vi "Update.vi"(8 "error in":errorcluster, 11 "Cobra GUI in":refnum<class "Cobra GUI.lvclass">) -> (0 "error out":errorcluster, 3 "Cobra GUI out":refnum<class "Cobra GUI.lvclass">)   [LabVIEW 2019, in "Cobra GUI.lvlib" / "Cobra GUI.lvclass"]
uses:
  Cobra GUI.lvclass
  GUI 1.0/Controls/Module Graphs.ctl
  GUI 1.0/GUI.lvlib
  GUI 1.0/Controls/System Graphs.ctl
  GUI 1.0/Controls/Gauge Graphs/Current.ctl
  GUI 1.0/Controls/Gauge Graphs/Superheat.ctl
  GUI 1.0/Controls/Gauge Graphs/Subcooling.ctl
  GUI 1.0/Controls/Gauge Graphs/Compression Ratio.ctl
  GUI 1.0/Controls/Dial Gauges.ctl
  07690957-dc4f-472d-b35f-df7a883bd9a6.vi
  4b12478f-287d-4315-ba79-d40235526ef4.vi
  Private Controls/Module Command.ctl
  2d39f8a6-1858-4a68-ac92-16f5d1316896.vi
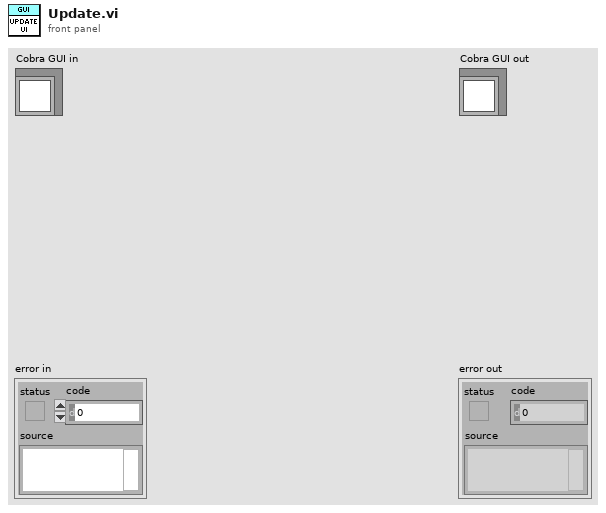
[diagram p1: front panel]
types:
  T1 = typedef "GUI.lvlib/System Graphs.ctl" = cluster{"Ambient Temp":dbl, "Suction Temp":dbl, "Condensor Temp":dbl, "Discharge Temp":dbl, "Bypass Steps":dbl}
  T2 = cluster{"M2 Thermal State":enum16{"Ramp Up", "Ramp Down", "Steady State", "Ebb and Flow", "Up", "Under Load", "Cryo Mode", "Shuttle Mode"}, "M1 Thermal State":enum16{"Ramp Up", "Ramp Down", "Steady State", "Ebb and Flow", "Up", "Under Load", "Cryo Mode"}, "High Side RPM":dbl, "Low Side RPM":dbl}
  T3 = typedef "GUI.lvlib/Dial Gauges.ctl" = cluster{"Condensing Pressure(psi)":dbl, "Compression Ratio":T4, "Subcool":T5, "Superheat":T6, "Current(A)":T7, "Suction Pressure(psi)":dbl}
  T4 = typedef "GUI.lvlib/Compression Ratio.ctl" = dbl
  T5 = typedef "GUI.lvlib/Subcooling.ctl" = dbl
  T6 = typedef "GUI.lvlib/Superheat.ctl" = dbl
  T7 = typedef "GUI.lvlib/Current.ctl" = dbl
  T8 = cluster{"Serial Number":string, "Compressor Hours":dbl, "SOM Storage(MB)":dbl, "Memory Available":dbl, "CPU Usage":dbl, "Software Version":string, "SD card free space":dbl, "Comp Temp":dbl, "Sleep Timer":dbl, "Sleep":bool, "Boot Up Time":timestamp}
  T9 = cluster{"M2 Heater %":dbl, "M2 Actuated":bool, "M2 Error":bool, "M2 Thermal Status":enum16{"Ramp Up", "Ramp Down", "Steady State", "Ebb and Flow", "Up", "Under Load", "Cryo Mode"}, "M2 Head State":enum16{"Disabled", "Run", "Error"}, "M2 Buffer":dbl, "M2 Valve Output":dbl}
  T10 = cluster{"M1 Heater %":dbl, "M1 Actuated":bool, "M1 Error":bool, "M1 Thermal Status":enum16{"Ramp Up", "Ramp Down", "Steady State", "Ebb and Flow", "Up", "Under Load", "Cryo Mode"}, "M1 Head State":enum16{"Disabled", "Run", "Error"}, "M1 Buffer":dbl, "M1 Valve Output":dbl}
  T11 = cluster{"Condensing Pressure":dbl, "Suction Pressure":dbl, "Bypass steps":u16, "Operating Time":dbl, "SubCooling":dbl, "Superheat":dbl, "M1 Superheat":dbl, "M2 Superheat":dbl, "Autotune output":dbl, "M1 Testing Elapsed Time":dbl, "M2 Testing Elapsed Time":dbl, "M1 Valve Control Mode":u8, "System Amps":dbl, "Compressor Run Time":dbl, "SD card free Space":dbl, "Free Memory":dbl, "M1 Pressure Feedback":dbl, "M2 Pressure Feedback":dbl, "Compression Ratio":dbl, "Serial Number":dbl, "M1 AC Load V":dbl, "M1 AC Load W":dbl, "M1 DC Load W":dbl, "M1 RH":dbl, "RH Threshold":dbl}
  T12 = cluster{"Name":string, "Time Stamp":timestamp, "Code":string, "Source":string, "Value":dbl, "Boolean":bool, "String":string, "Error":bool, "Warning":bool, " Fault":bool}[]
  T13 = cluster{"High Stage manual speed control":bool, "Manual High stage frequency":dbl, "Low Stage manual speed control":bool, "Manual Low Stage frequency":dbl}
  T14 = enum16{"Sleeping", "Warming up", "Ready", "Testing", "Restless", "Idle", "Sleeping Fault", "warning"}
  T15 = cluster{"port ":u16, "remote address":string, "Connection timeout ms":i32, "Waiting for connection":bool, "Waiting for Command":bool, "timeout ms":i32}[]
  T16 = typedef "LabGUI.lvlib/Module Command.ctl" = cluster{"Set Temp":dbl[unit], "Read Temp":dbl[unit], "Package":u16, "Bin String":string, "M1 Enable":bool, "TSD":bool}
  T17 = typedef "GUI.lvlib/System Status.ctl" = cluster{"Power On Off":bool, "Discharge Temp":dbl, "Liquid Temp":dbl, "Suction Temp":dbl, "Ambient Temp":dbl, "Sleep":bool, "System Status":u16, "M1 Actuated":bool, "M2 Actuated":bool, "Sleep Timer":dbl, "M1 Bin":cluster{"Bin String":string, "Bin Color":u16}, "M2 Bin":cluster{"Bin String":string, "Bin Color":u16}, "Discharge Pressure":dbl, "Suction Pressure":dbl, "Compression Ratio":dbl, "Compressor Amps":dbl, "Compressor Hours":dbl, "Bypass Steps":u16, "SubCooling":dbl, "SuperHeat":dbl, "Serial Number":string, "EMO detected":bool, "EMO Tripped":bool, "Thermal cutoff":bool, "Thermal cutoff 2":bool, "High Pressure switch":bool, "Running Time":timestamp, "SOM Status":cluster{"Boot Up Time":timestamp, "Software Version":string, "CPU Usage":dbl, "Memory Available":dbl, "SD card free space":dbl, "SOM Storage":dbl}, "Cascade Extra":cluster{"Discharge Temp High Side":dbl, "Suction Temp High Side":dbl, "Liquid Temp High side":dbl, "Discharge Pressure 2":dbl, "Suction Pressure 2":dbl, "Low Side RPM":dbl, "High Side RPM":dbl}}
  T18 = typedef "GUI.lvlib/Module Status.ctl" = cluster{"Case Temp":dbl, "Evap Temp":dbl, "Heater %":dbl, "EEV Steps":u32, "Set Temp":dbl, "Feedback":u8, "Power Drive":bool, "Piston Volts":dbl, "Safe Temp":bool, "Power":bool, "Thermal State":u16, "Error":bool, "In tollerance":bool, "Head State":u16, "Piston Force":dbl, "Package":string, "Dynamic SV":dbl, "PV":dbl, "TSD Temp":dbl, "DC Load Watts":dbl, "AC Load Watts":dbl, "Intec Feedback":dbl}
  T19 = typedef "GUI.lvlib/Config Data.ctl" = cluster{"Packages":cluster{"DUT Force lbf":cluster{" 0":u32, " 1":u32, " 2":u32, "3":u32, "4":u32, "5":u32, " 6":u32, "7":u32, "8":u32, "9":u32}, "DUT Names":cluster{"0":string, "1":string, "2":string, "3":string, "4":string, "5":string, "6":string, "7":string, "8":string, "9":string}}, "Heater PID":cluster{"P":dbl, "I":dbl, "D":dbl}, "Piston Settings":cluster{"Forces Slope":dbl, "Forces Intercept":dbl, "Transition Force":dbl, "Up Force":dbl, "Diameter (mm)":dbl, "Delay (ms)":dbl, "Pressure Ramp Delay (ms)":dbl}, "Safe Temps":cluster{"Minimum":i32, "Enabled":bool, "Maximum":i32}, "System Settings":cluster{"Number of Heads":i32, "60Hz Power":bool, "FTC200":bool, "AutoStartup":bool, "Purge":bool, "Sensors":bool, "HandClamp":bool, "ATE":bool, "Benchtop":bool, "Production":bool, "Refrigerant":u16, "Handler":bool, "Shuttle":bool, "220V":bool, "Cascade":bool, "Suction Sensor":u16, "Discharge Sensor":u16}, "Stepper Settings ":cluster{"Microstepping":u16, "Velocity":u8}, "Set Point Range":cluster{"Max":dbl, "Min":dbl}, "Pedestal Check DeltaT":dbl, "Ramp Delta T":dbl, "Ramp-SS Threshold":dbl, "SS Tolerance":dbl, "EEV PID":cluster{"Ramp Up Target":dbl, "Ramp Down Target":dbl, "Steady State Target":dbl, "Output":cluster{"Max":dbl, "Min":dbl}, "EBB and Flow Temp TH":dbl, "Cryomode EEV Max":dbl, "Valve minimum opening ":dbl, "Ramp Up EEV Steps":dbl, "Ramp Down EEV Steps":dbl, "SS EEV Steps Reset":dbl, "EBB and Flow Tol":dbl, "Gains":cluster{"P":dbl, "I":dbl, "D":dbl}, "Dissabled Target":dbl, "CryoMode Gains":cluster{"P":dbl, "I":dbl, "D":dbl}, "M1 SuperHeat Setpoint":dbl, "M2 Gains":cluster{"P":dbl, "I":dbl, "D":dbl}, "Flow Curve":u16}, "Sleep Timeout":dbl, "Bypass Values":cluster{"Bypass Valve":bool, "Flow Curve":u16, "Output":cluster{"Max":u32, "Min":u32}, "Feedback":u16, "Cyth Bypass":bool, "PID":cluster{"P":dbl, "I":dbl, "D":dbl}, "Pressure setpoint":i16, "Cryo Temp":i16, "Superheat Setpoint":i16, "Cryo Setpoint":i16}, "Default Temp":dbl, "InTEC":cluster{"Enabled":bool, "IP":string, "Port":u16}, "M1 TSD":cluster{"Gain":dbl, "Offset":dbl, "V Offset ":dbl}, "M2 TSD":cluster{"Gain":dbl, "Offset":dbl, "V Offset ":dbl}, "M1 T-Case Calibration":cluster{"Gain":dbl, "Offset":dbl}, "M2 T-Case Calibration":cluster{"Gain":dbl, "Offset":dbl}, "Heater PID TSD":cluster{"P":dbl, "I":dbl, "D":dbl}, "M2 Heater PID":cluster{"P":dbl, "I":dbl, "D":dbl}}
  T20 = cluster{"Compressor:":refnum<vi>, "NS Connection":refnum<vi>, "M1 Graphs":refnum<vi>, "M1 Main Waveform":refnum<vi>, "M2 Main Waveform":refnum<vi>, "M1 State":refnum<vi>, "M2 State":refnum<vi>, "M1 Commands":refnum<vi>, "M2 Commands":refnum<vi>, "M2 Graphs":refnum<vi>, "System Graphs":refnum<vi>, "M1 Cluster":refnum<vi>, "M2 Cluster":refnum<vi>, "TCP Connections":refnum<vi>, "M1 Humidity":refnum<vi>, "RT Status":refnum<vi>, "M1 Safe Temp and Head State":refnum<vi>, "M2 Safe Temp and Head State":refnum<vi>, "M1 Power Drive":refnum<vi>, "M2 Power Drive":refnum<vi>, "Gauges":refnum<vi>, "Cascade Compressor controls":refnum<vi>, "TCP commands":refnum<vi>, "Errors":refnum<vi>, "RT Events":refnum<vi>, "System Cluster":refnum<vi>, "Power On-Off":refnum<vi>, "Thermal Info":refnum<vi>, "Connected System":refnum<vi>}
  T21 = cluster{"Set Temp":dbl, "Read Temp":dbl, "Package":string, "Force":dbl, "Feedback":u8}
  T22 = cluster{"Set Temp":dbl[unit], "Read Temp":dbl[unit], "Package":u16, "Bin String":string, "M Enable":bool, "TSD":bool}
  T23 = cluster{"0":string, "1":string, "2":string, "3":string, "4":string, "5":string, "6":string, "7":string, "8":string, "9":string}
  T24 = typedef "GUI.lvlib/Module Graphs.ctl" = cluster{"Case Temp":dbl, "Evap Temp":dbl, "Heater Power (%)":dbl, "EEV Steps":dbl, "AC Load(W)":dbl}
  T25 = cluster{"Heater %":dbl, "Actuated":bool, "Error":bool, "Thermal Status":enum16{"Ramp Up", "Ramp Down", "Steady State", "Ebb and Flow", "Up", "Under Load", "Cryo Mode"}, "Head State":enum16{"Disabled", "Run", "Error"}, "Buffer":dbl, "Valve Output":dbl}
  T26 = cluster{"Boot Up Time":timestamp, "Software Version":string, "CPU Usage":dbl, "Memory Available":dbl, "SD card free space":dbl, "SOM Storage":dbl}
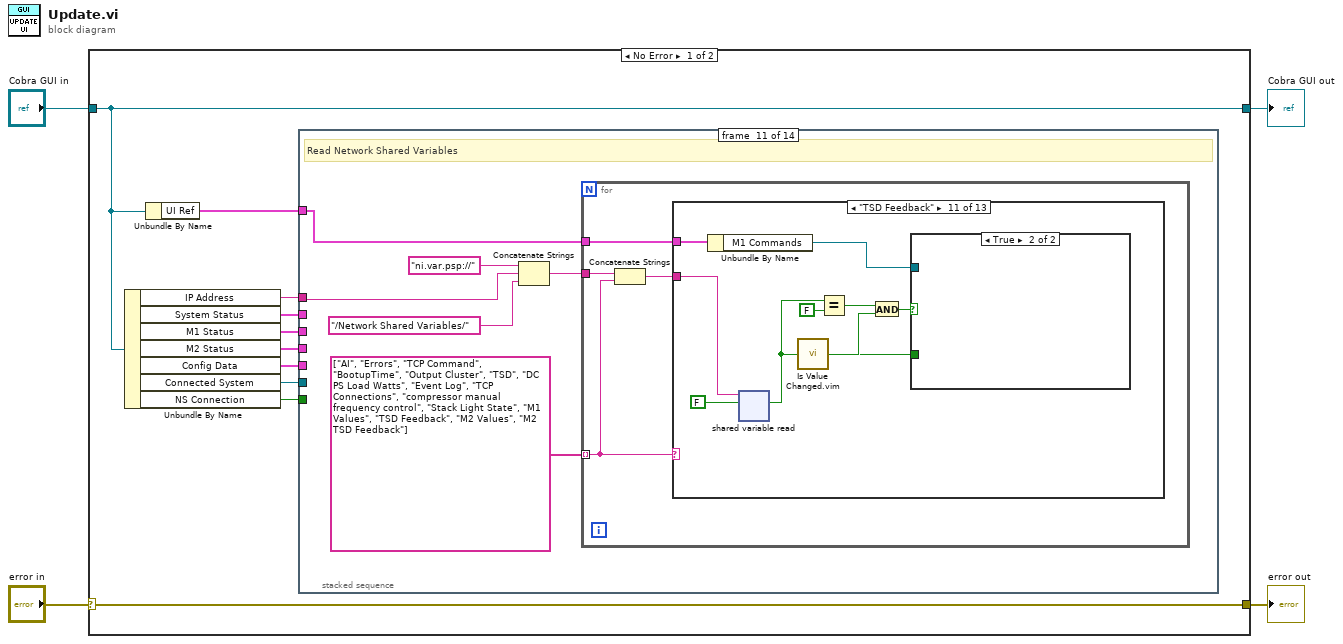
[diagram p0: block diagram]
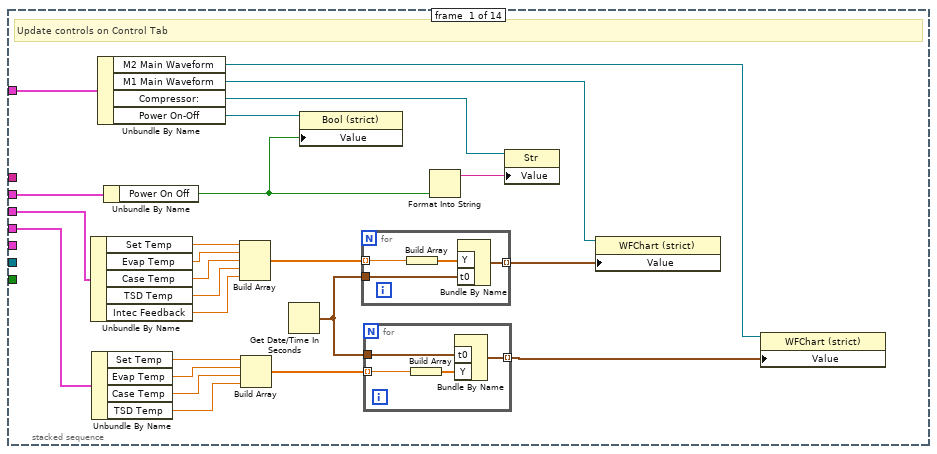
[diagram p2: hidden frame]
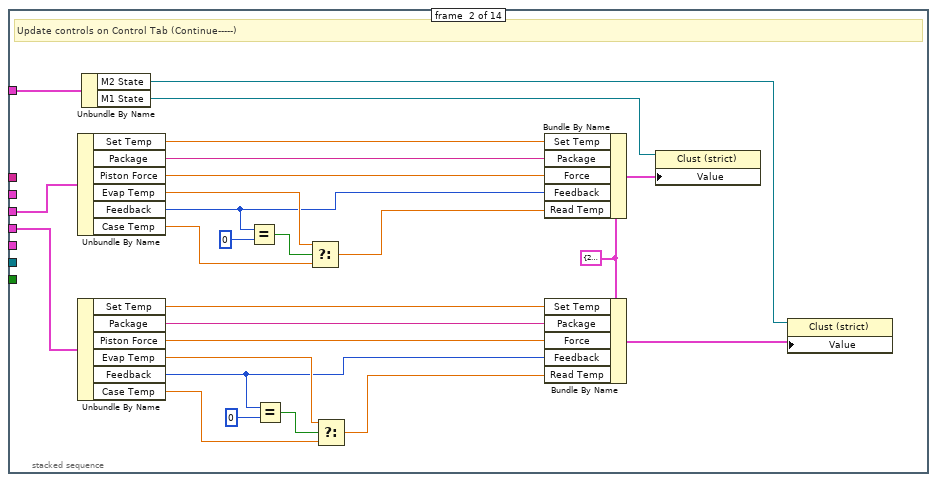
[diagram p3: hidden frame]
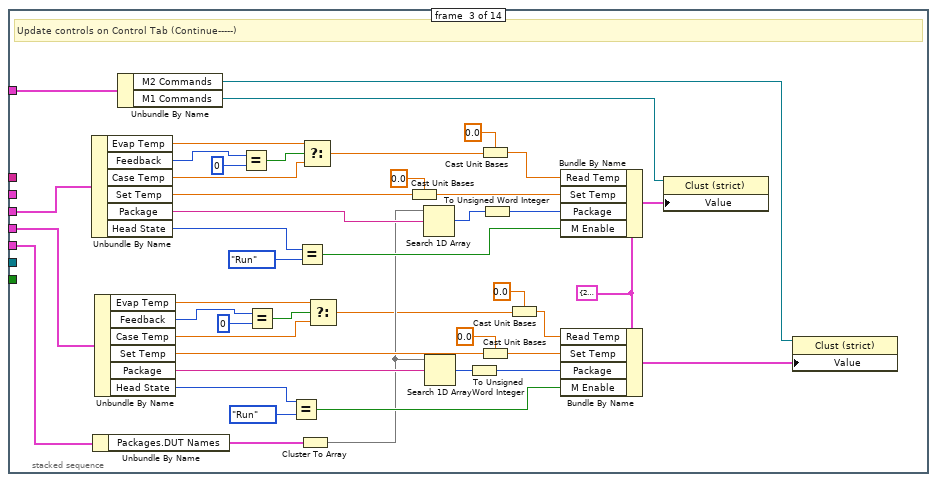
[diagram p4: hidden frame]
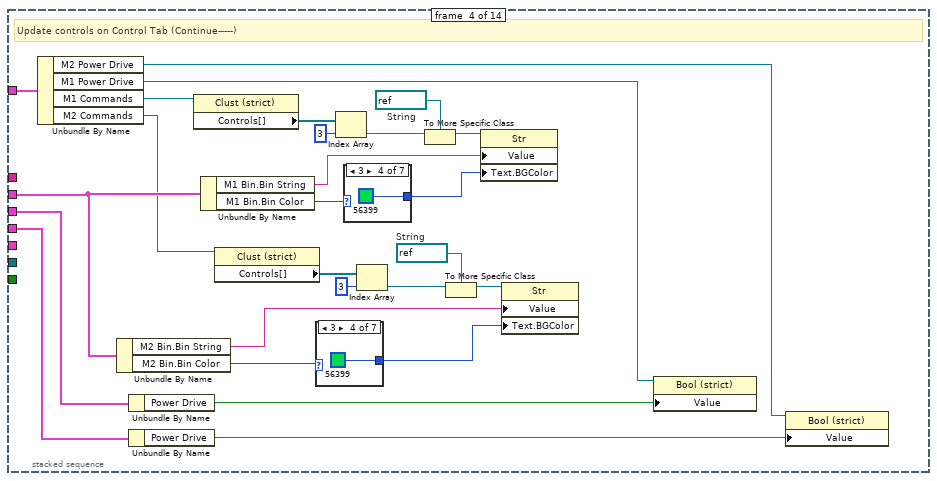
[diagram p5: hidden frame]
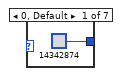
[diagram p6: hidden frame]
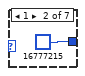
[diagram p7: hidden frame]
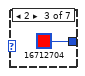
[diagram p8: hidden frame]
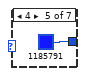
[diagram p9: hidden frame]
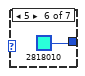
[diagram p10: hidden frame]
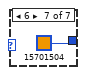
[diagram p11: hidden frame]
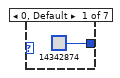
[diagram p12: hidden frame]
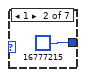
[diagram p13: hidden frame]
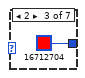
[diagram p14: hidden frame]
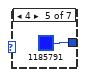
[diagram p15: hidden frame]
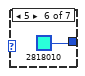
[diagram p16: hidden frame]
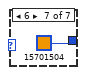
[diagram p17: hidden frame]
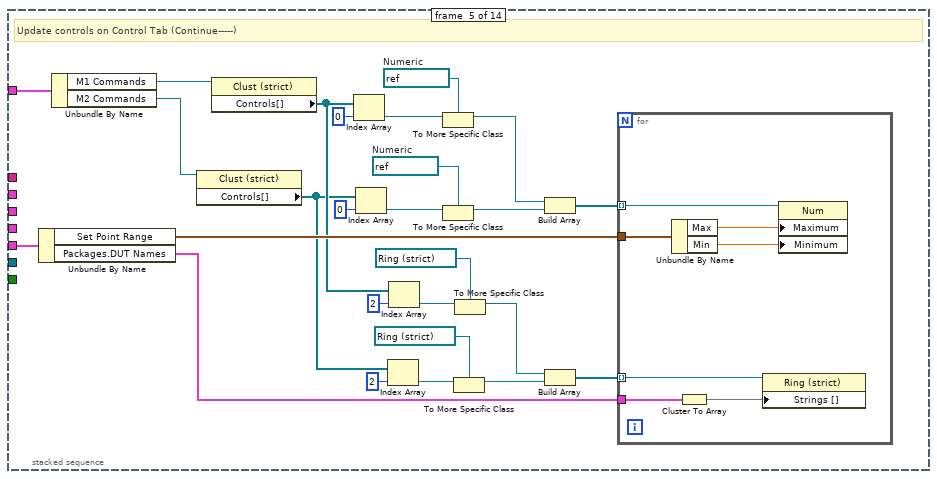
[diagram p18: hidden frame]
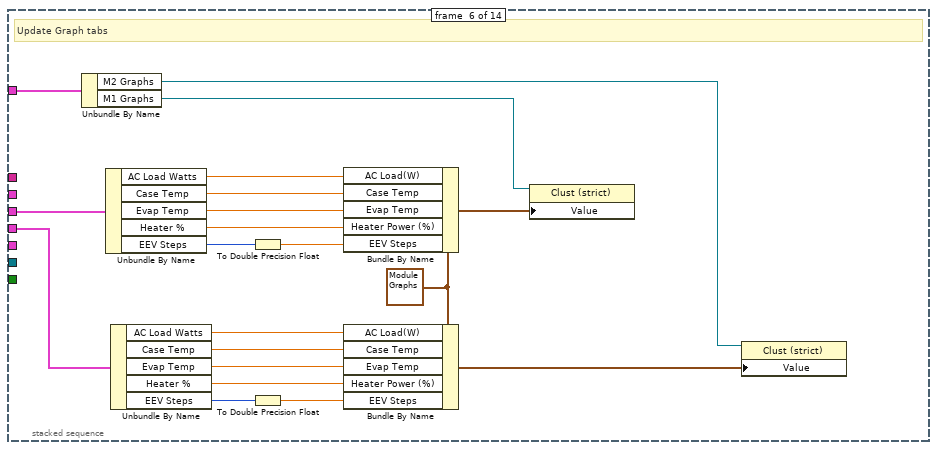
[diagram p19: hidden frame]
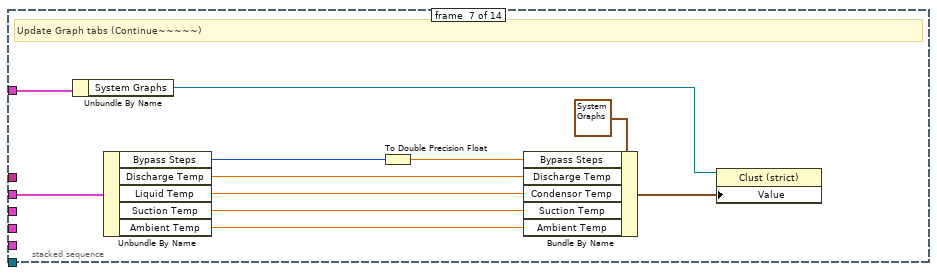
[diagram p20: hidden frame]
diagram:
  n1 = case shown="No Error" "error in" {
    selector: "error in" -> [w14 w440]
    tunnel: [w14 w440] -> w3
    tunnel: [w13 w439] -> w1
    tunnel: "Cobra GUI in" -> [w13 w439]
    frame No Error {
      n2 = Unbundle By Name(w13) -> ("IP Address"=w12:string, "System Status"=w11:T17, "M1 Status"=w10:T18, "M2 Status"=w9:T18, "Config Data"=w8:T19, "Connected System"=w7:refnum<vi>, "NS Connection"=w6:bool)
      n3 = Unbundle By Name(w13) -> ("UI Ref"=w5:T20)
      n4 = stacked-sequence {
        tunnel: w12 -> [_ _ _ _ _ _ _ _ _ _ w299 _ _ _]
        tunnel: w11 -> [w19 _ _ w143 _ _ w214 w229 w253 w292 _ _ _ w438]
        tunnel: w10 -> [w26 w57 w96 w142 _ w196 _ w228 w252 _ _ w411 _ _]
        tunnel: w9 -> [w25 w56 w95 w141 _ w195 _ w227 w251 _ _ _ w412 _]
        tunnel: w8 -> [_ _ w94 _ w183 _ _ _ _ _ _ w405 w419 w437]
        tunnel: w7 -> [_ _ _ _ _ _ _ _ _ _ _ _ _ _]
        tunnel: w6 -> [_ _ _ _ _ _ _ _ _ _ _ _ _ _]
        tunnel: w5 -> [w24 w55 w93 w140 w182 w197 w213 w226 w250 w279 w296 w410 w424 w431]
        frame #0 {
          # "Update controls on Control Tab"
          n5 = Unbundle By Name(w26) -> ("Set Temp"=w28:dbl, "Evap Temp"=w29:dbl, "Case Temp"=w30:dbl, "TSD Temp"=w31:dbl, "Intec Feedback"=w32:dbl)
          n6 = Unbundle By Name(w25) -> ("Set Temp"=w34:dbl, "Evap Temp"=w35:dbl, "Case Temp"=w36:dbl, "TSD Temp"=w37:dbl)
          n7 = Unbundle By Name(w24) -> ("M2 Main Waveform"=w20:refnum<vi>, "M1 Main Waveform"=w23:refnum<vi>, "Compressor:"=w18:refnum<vi>, "Power On-Off"=w16:refnum<vi>)
          n8 = Unbundle By Name(w19) -> ("Power On Off"=w15:bool)
          n9 = Build Array(w28, w29, w30, w31, w32) -> (w33:dbl[])
          n10 = Build Array(w34, w35, w36, w37) -> (w38:dbl[])
          n11 = Get Date/Time In Seconds() -> (seconds since 1Jan1904=w27:timestamp)
          n12 = property class="Bool (strict)"(reference=w16, "Value"=w15) -> ()  [unwired: 1 in, 2 out]
          n13 = for {
            tunnel: [w42] -> w22 mode=indexing
            tunnel: w27 -> [w41]
            tunnel: w33 -> [w39] mode=indexing
            n14 = Build Array(w39) -> (w40:dbl[])
            n15 = Bundle By Name("Y"=w40, "t0"=w41) -> (w42:waveform(dbl))  [unwired: 1 in]
          }
          n16 = for {
            tunnel: w27 -> [w45]
            tunnel: [w46] -> w21 mode=indexing
            tunnel: w38 -> [w43] mode=indexing
            n17 = Build Array(w43) -> (w44:dbl[])
            n18 = Bundle By Name("t0"=w45, "Y"=w44) -> (w46:waveform(dbl))  [unwired: 1 in]
          }
          n19 = Format Into String(w15) -> (resulting string=w17:string)  [unwired: 3 in, 1 out]
          n20 = property class="Str"(reference=w18, "Value"=w17) -> ()  [unwired: 1 in, 2 out]
          n21 = property class="WFChart (strict)"(reference=w23, "Value"=w22) -> ()  [unwired: 1 in, 2 out]
          n22 = property class="WFChart (strict)"(reference=w20, "Value"=w21) -> ()  [unwired: 1 in, 2 out]
        }
        frame #1 {
          w58 = T21 {"Set Temp"=20.0, "Read Temp"=0.0, "Package"="", "Force"=0.0, "Feedback"=1} ("M2 Data")
          # "Update controls on Control Tab (Continue-----)"
          n23 = Unbundle By Name(w57) -> ("Set Temp"=w59:dbl, "Package"=w60:string, "Piston Force"=w61:dbl, "Evap Temp"=w64:dbl, "Feedback"=w47:u8, "Case Temp"=w65:dbl)
          n24 = Unbundle By Name(w56) -> ("Set Temp"=w66:dbl, "Package"=w67:string, "Piston Force"=w68:dbl, "Evap Temp"=w72:dbl, "Feedback"=w49:u8, "Case Temp"=w71:dbl)
          n25 = Unbundle By Name(w55) -> ("M2 State"=w51:refnum<vi>, "M1 State"=w54:refnum<vi>)
          n26 = Equal?(x=w47, y=u8 0) -> (x = y?=w62:bool)
          n27 = Equal?(x=w49, y=u8 0) -> (x = y?=w70:bool)
          n28 = Select(t=w64, s=w62, f=w65) -> (s? t:f=w48:dbl)
          n29 = Select(t=w72, s=w70, f=w71) -> (s? t:f=w50:dbl)
          n30 = Bundle By Name(cluster=w58, "Set Temp"=w59, "Package"=w60, "Force"=w61, "Feedback"=w47, "Read Temp"=w48) -> (w53:T21)
          n31 = Bundle By Name(cluster=w58, "Set Temp"=w66, "Package"=w67, "Force"=w68, "Feedback"=w49, "Read Temp"=w50) -> (w52:T21)
          n32 = property on="Property Node" class="Clust (strict)"(reference=w54, "Value"=w53) -> ()  [unwired: 1 in, 2 out]
          n33 = property on="Property Node" class="Clust (strict)"(reference=w51, "Value"=w52) -> ()  [unwired: 1 in, 2 out]
        }
        frame #2 {
          w97 = T22 {"Set Temp"=273.15, "Read Temp"=273.15, "Package"=0, "Bin String"="", "M Enable"=TRUE, "TSD"=TRUE} ("M1 Commands")
          # "Update controls on Control Tab (Continue-----)"
          n34 = Unbundle By Name(w96) -> ("Evap Temp"=w82:dbl, "Feedback"=w83:u8, "Case Temp"=w84:dbl, "Set Temp"=w112:dbl, "Package"=w100:string, "Head State"=w103:u16)
          n35 = Unbundle By Name(w94) -> ("Packages.DUT Names"=w99:T23)
          n36 = Unbundle By Name(w95) -> ("Evap Temp"=w74:dbl, "Feedback"=w75:u8, "Case Temp"=w76:dbl, "Set Temp"=w115:dbl, "Package"=w101:string, "Head State"=w105:u16)
          n37 = Unbundle By Name(w93) -> ("M2 Commands"=w90:refnum<vi>, "M1 Commands"=w91:refnum<vi>)
          n38 = Equal?(x=w83, y=u8 0) -> (x = y?=w87:bool)
          n39 = Equal?(x=w75, y=u8 0) -> (x = y?=w78:bool)
          n40 = Equal?(x=w105, y=enum16{"Disabled", "Run", "Error"}."Run" ("Dataset.M1 Status.Head State")) -> (x = y?=w108:bool)
          n41 = Equal?(x=w103, y=enum16{"Disabled", "Run", "Error"}."Run" ("Dataset.M1 Status.Head State")) -> (x = y?=w111:bool)
          n42 = Cluster To Array(cluster=w99) -> (array=w98:string[])
          n43 = Select(t=w82, s=w87, f=w84) -> (s? t:f=w88:dbl)
          n44 = Select(t=w74, s=w78, f=w76) -> (s? t:f=w77:dbl)
          n45 = Cast Unit Bases(0:w112, 1:dbl[unit] 0.0 ("Set Temp")) -> (2:w113:dbl[unit])
          n46 = Search 1D Array(1D array=w98, element=w100) -> (index of element=w109:i32)  [unwired: 1 in]
          n47 = Search 1D Array(1D array=w98, element=w101) -> (index of element=w106:i32)  [unwired: 1 in]
          n48 = To Unsigned Word Integer(number=w106) -> (unsigned 16bit integer=w107:u16)
          n49 = Cast Unit Bases(0:w88, 1:dbl[unit] 0.0 ("Value")) -> (2:w81:dbl[unit])
          n50 = Cast Unit Bases(0:w115, 1:dbl[unit] 0.0 ("Set Temp")) -> (2:w117:dbl[unit])
          n51 = To Unsigned Word Integer(number=w109) -> (unsigned 16bit integer=w110:u16)
          n52 = Cast Unit Bases(0:w77, 1:dbl[unit] 0.0 ("Value")) -> (2:w73:dbl[unit])
          n53 = Bundle By Name(cluster=w97, "Read Temp"=w81, "Set Temp"=w113, "Package"=w110, "M Enable"=w111) -> (w92:T22)
          n54 = Bundle By Name(cluster=w97, "Read Temp"=w73, "Set Temp"=w117, "Package"=w107, "M Enable"=w108) -> (w89:T22)
          n55 = property on="Property Node" class="Clust (strict)"(reference=w91, "Value"=w92) -> ()  [unwired: 1 in, 2 out]
          n56 = property on="Property Node" class="Clust (strict)"(reference=w90, "Value"=w89) -> ()  [unwired: 1 in, 2 out]
        }
        frame #3 {
          w124 = refnum<vi> refnum  # String
          w130 = refnum<vi> refnum  # String
          # "Update controls on Control Tab (Continue-----)"
          n57 = Unbundle By Name(w140) -> ("M2 Power Drive"=w136:refnum<vi>, "M1 Power Drive"=w138:refnum<vi>, "M1 Commands"=w139:refnum<vi>, "M2 Commands"=w118:refnum<vi>)
          n58 = Unbundle By Name(w143) -> ("M2 Bin.Bin String"=w119:string, "M2 Bin.Bin Color"=w134:u16)
          n59 = Unbundle By Name(w142) -> ("Power Drive"=w137:bool)
          n60 = Unbundle By Name(w141) -> ("Power Drive"=w135:bool)
          n61 = property class="Clust (strict)"(reference=w139) -> ("Controls[]"=w133:refnum<vi>[])  [unwired: 1 in, 2 out]
          n62 = Unbundle By Name(w143) -> ("M1 Bin.Bin String"=w128:string, "M1 Bin.Bin Color"=w127:u16)
          n63 = property class="Clust (strict)"(reference=w118) -> ("Controls[]"=w121:refnum<vi>[])  [unwired: 1 in, 2 out]
          n64 = case shown="3" w134 {
            tunnel: [u32 14342874 u32 16777215 u32 16712704 u32 56399 u32 1185791 u32 2818010 u32 15701504] -> w120
            frame 0, Default {
            }
            frame 1 {
            }
            frame 2 {
            }
            frame 3 {
            }
            frame 4 {
            }
            frame 5 {
            }
            frame 6 {
            }
          }
          n65 = Index Array(array=w133, index=3) -> (element=w132:refnum<vi>)
          n66 = case shown="3" w127 {
            tunnel: [u32 14342874 u32 16777215 u32 16712704 u32 56399 u32 1185791 u32 2818010 u32 15701504] -> w126
            frame 0, Default {
            }
            frame 1 {
            }
            frame 2 {
            }
            frame 3 {
            }
            frame 4 {
            }
            frame 5 {
            }
            frame 6 {
            }
          }
          n67 = Index Array(array=w121, index=3) -> (element=w122:refnum<vi>)
          n68 = To More Specific Class(target class=w130, reference=w132) -> (specific class reference=w129:refnum<vi>)  [unwired: 1 in, 1 out]
          n69 = To More Specific Class(target class=w124, reference=w122) -> (specific class reference=w125:refnum<vi>)  [unwired: 1 in, 1 out]
          n70 = property class="Str"(reference=w129, "Value"=w128, "Text.BGColor"=w126) -> ()  [unwired: 1 in, 2 out]
          n71 = property class="Str"(reference=w125, "Value"=w119, "Text.BGColor"=w120) -> ()  [unwired: 1 in, 2 out]
          n72 = property class="Bool (strict)"(reference=w138, "Value"=w137) -> ()  [unwired: 1 in, 2 out]
          n73 = property class="Bool (strict)"(reference=w136, "Value"=w135) -> ()  [unwired: 1 in, 2 out]
        }
        frame #4 {
          w169 = refnum<vi> refnum  # Numeric
          w176 = refnum<vi> refnum  # Numeric
          # "Update controls on Control Tab (Continue-----)"
          n74 = Unbundle By Name(w183) -> ("Set Point Range"=w181:cluster{"Max":dbl, "Min":dbl}, "Packages.DUT Names"=w180:T23)
          n75 = Unbundle By Name(w182) -> ("M1 Commands"=w177:refnum<vi>, "M2 Commands"=w175:refnum<vi>)
          n76 = property class="Clust (strict)"(reference=w175) -> ("Controls[]"=w160:refnum<vi>[])  [unwired: 1 in, 2 out]
          n77 = property class="Clust (strict)"(reference=w177) -> ("Controls[]"=w166:refnum<vi>[])  [unwired: 1 in, 2 out]
          n78 = Index Array(array=w166, index=0) -> (element=w179:refnum<vi>)
          n79 = Index Array(array=w160, index=0) -> (element=w173:refnum<vi>)
          n80 = Index Array(array=w160, index=2) -> (element=w162:refnum<vi>)
          n81 = Index Array(array=w166, index=2) -> (element=w167:refnum<vi>)
          n82 = To More Specific Class(target class=w176, reference=w179) -> (specific class reference=w172:refnum<vi>)  [unwired: 1 in, 1 out]
          n83 = To More Specific Class(target class=w169, reference=w173) -> (specific class reference=w171:refnum<vi>)  [unwired: 1 in, 1 out]
          n84 = To More Specific Class(target class=refnum<vi> refnum ("Package"), reference=w162) -> (specific class reference=w159:refnum<vi>)  [unwired: 1 in, 1 out]
          n85 = To More Specific Class(target class=refnum<vi> refnum ("Package"), reference=w167) -> (specific class reference=w164:refnum<vi>)  [unwired: 1 in, 1 out]
          n86 = Build Array(w172, w171) -> (w170:refnum<vi>[])
          n87 = Build Array(w164, w159) -> (w158:refnum<vi>[])
          n88 = for {
            tunnel: w170 -> [w188] mode=indexing
            tunnel: w181 -> [w187]
            tunnel: w180 -> [w185]
            tunnel: w158 -> [w186] mode=indexing
            n89 = Unbundle By Name(w187) -> ("Max"=w189:dbl, "Min"=w190:dbl)
            n90 = Cluster To Array(cluster=w185) -> (array=w184:string[])
            n91 = property class="Ring (strict)"(reference=w186, "Strings []"=w184) -> ()  [unwired: 1 in, 2 out]
            n92 = property class="Num"(reference=w188, "Maximum"=w189, "Minimum"=w190) -> ()  [unwired: 1 in, 2 out]
          }
        }
        frame #5 {
          w210 = T24 {"Case Temp"=24.9375, "Evap Temp"=24.8046875, "Heater Power (%)"=0.0, "EEV Steps"=0.0, "AC Load(W)"=10.492394664499656} ("M1 Graphs")
          # "Update Graph tabs"
          n93 = Unbundle By Name(w197) -> ("M2 Graphs"=w192:refnum<vi>, "M1 Graphs"=w194:refnum<vi>)
          n94 = Unbundle By Name(w196) -> ("AC Load Watts"=w198:dbl, "Case Temp"=w199:dbl, "Evap Temp"=w200:dbl, "Heater %"=w201:dbl, "EEV Steps"=w202:u32)
          n95 = Unbundle By Name(w195) -> ("AC Load Watts"=w204:dbl, "Case Temp"=w205:dbl, "Evap Temp"=w206:dbl, "Heater %"=w207:dbl, "EEV Steps"=w208:u32)
          n96 = To Double Precision Float(number=w202) -> (double precision float=w203:dbl)
          n97 = To Double Precision Float(number=w208) -> (double precision float=w209:dbl)
          n98 = Bundle By Name(cluster=w210, "AC Load(W)"=w198, "Case Temp"=w199, "Evap Temp"=w200, "Heater Power (%)"=w201, "EEV Steps"=w203) -> (w193:T24)
          n99 = Bundle By Name(cluster=w210, "AC Load(W)"=w204, "Case Temp"=w205, "Evap Temp"=w206, "Heater Power (%)"=w207, "EEV Steps"=w209) -> (w191:T24)
          n100 = property class="Clust (strict)"(reference=w194, "Value"=w193) -> ()  [unwired: 1 in, 2 out]
          n101 = property class="Clust (strict)"(reference=w192, "Value"=w191) -> ()  [unwired: 1 in, 2 out]
        }
        frame #6 {
          # "Update Graph tabs (Continue~~~~~)"
          n102 = Unbundle By Name(w213) -> ("System Graphs"=w212:refnum<vi>)
          n103 = Unbundle By Name(w214) -> ("Bypass Steps"=w216:u16, "Discharge Temp"=w218:dbl, "Liquid Temp"=w219:dbl, "Suction Temp"=w220:dbl, "Ambient Temp"=w221:dbl)
          n104 = To Double Precision Float(number=w216) -> (double precision float=w217:dbl)
          n105 = Bundle By Name(cluster=T1 {"Ambient Temp"=77.534379824996, "Suction Temp"=77.78750485181808, "Condensor Temp"=77.29531729966402, "Discharge Temp"=78.09687988460064, "Bypass Steps"=72.0} ("System Graphs"), "Bypass Steps"=w217, "Discharge Temp"=w218, "Condensor Temp"=w219, "Suction Temp"=w220, "Ambient Temp"=w221) -> (w211:T1)
          n106 = property class="Clust (strict)"(reference=w212, "Value"=w211) -> ()  [unwired: 1 in, 2 out]
        }
        frame #7 {
          # "Update Graph tabs (Continue~~~~~)"
          n107 = Unbundle By Name(w226) -> ("Thermal Info"=w223:refnum<vi>, "Gauges"=w225:refnum<vi>)
          n108 = Unbundle By Name(w229) -> ("Compression Ratio"=w231:dbl, "Compressor Amps"=w232:dbl, "Discharge Pressure"=w233:dbl, "Suction Pressure"=w234:dbl, "SubCooling"=w235:dbl, "SuperHeat"=w236:dbl, "Cascade Extra.High Side RPM"=w240:dbl, "Cascade Extra.Low Side RPM"=w241:dbl)
          n109 = Unbundle By Name(w228) -> ("Thermal State"=w238:u16)
          n110 = Unbundle By Name(w227) -> ("Thermal State"=w239:u16)
          n111 = Round To Nearest(number=w240) -> (nearest integer value=w242:dbl)
          n112 = Round To Nearest(number=w241) -> (nearest integer value=w243:dbl)
          n113 = Bundle By Name(cluster=T3 {"Condensing Pressure(psi)"=165.57116807812622, "Compression Ratio"=1.0119646390563775, "Subcool"=-0.3368072880168427, "Superheat"=1.4200558413526494, "Current(A)"=0.2333286882987343, "Suction Pressure(psi)"=163.4397897916897} ("Gauges"), "Compression Ratio"=w231, "Current(A)"=w232, "Condensing Pressure(psi)"=w233, "Suction Pressure(psi)"=w234, "Subcool"=w235, "Superheat"=w236) -> (w224:T3)
          n114 = Bundle By Name(cluster=T2 {"M2 Thermal State"=enum."Ramp Up", "M1 Thermal State"=enum."Steady State", "High Side RPM"=0.0, "Low Side RPM"=0.0} ("Thermal Info"), "High Side RPM"=w242, "Low Side RPM"=w243, "M1 Thermal State"=w238, "M2 Thermal State"=w239) -> (w222:T2)
          n115 = property class="Clust (strict)"(reference=w225, "Value"=w224) -> ()  [unwired: 1 in, 2 out]
          n116 = property class="Clust (strict)"(reference=w223, "Value"=w222) -> ()  [unwired: 1 in, 2 out]
        }
        frame #8 {
          w268 = T25 {"Heater %"=0.0, "Actuated"=FALSE, "Error"=FALSE, "Thermal Status"=enum."Steady State", "Head State"=enum."Disabled", "Buffer"=0.9999999999999998, "Valve Output"=0.0} ("M1 Cluster")
          # "Update Debug tab"
          n117 = Unbundle By Name(w250) -> ("M2 Cluster"=w245:refnum<vi>, "M1 Cluster"=w247:refnum<vi>, "System Cluster"=w249:refnum<vi>)
          n118 = Unbundle By Name(w253) -> ("Sleep"=w255:bool, "Sleep Timer"=w256:dbl, "Discharge Temp"=w257:dbl, "Compressor Hours"=w258:dbl, "Serial Number"=w259:string)
          n119 = Unbundle By Name(w252) -> ("Head State"=w260:u16, "Thermal State"=w261:u16, "Error"=w262:bool, "Heater %"=w263:dbl)
          n120 = Unbundle By Name(w251) -> ("Head State"=w264:u16, "Thermal State"=w265:u16, "Error"=w266:bool, "Heater %"=w267:dbl)
          n121 = Bundle By Name(cluster=T8 {"Serial Number"="204300076", "Compressor Hours"=59.65, "SOM Storage(MB)"=243.036, "Memory Available"=353.72, "CPU Usage"=40.953570959266244, "Software Version"="SW Version:CC 21.4.8.1", "SD card free space"=31.886, "Comp Temp"=78.09687988460064, "Sleep Timer"=-1.0, "Sleep"=TRUE, "Boot Up Time"=timestamp(3700144843.654765 s since 1904-01-01)} ("System Cluster"), "Sleep"=w255, "Sleep Timer"=w256, "Comp Temp"=w257, "Compressor Hours"=w258, "Serial Number"=w259) -> (w248:T8)
          n122 = Bundle By Name(cluster=w268, "Head State"=w260, "Thermal Status"=w261, "Error"=w262, "Heater %"=w263) -> (w246:T25)
          n123 = Bundle By Name(cluster=w268, "Head State"=w264, "Thermal Status"=w265, "Error"=w266, "Heater %"=w267) -> (w244:T25)
          n124 = property class="Clust (strict)"(reference=w249, "Value"=w248) -> ()  [unwired: 1 in, 2 out]
          n125 = property class="Clust (strict)"(reference=w247, "Value"=w246) -> ()  [unwired: 1 in, 2 out]
          n126 = property class="Clust (strict)"(reference=w245, "Value"=w244) -> ()  [unwired: 1 in, 2 out]
        }
        frame #9 {
          # "Update Debug tab (Continue~~~~)"
          n127 = Unbundle By Name(w279) -> ("System Cluster"=w278:refnum<vi>, "M2 Cluster"=w274:refnum<vi>, "M2 Cluster"=w272:refnum<vi>)
          n128 = Unbundle By Name(w292) -> ("M2 Actuated"=w269:bool, "M1 Actuated"=w273:bool, "SOM Status"=w280:T26)
          n129 = Unbundle By Name(w280) -> ("Memory Available"=w283:dbl, "SOM Storage"=w284:dbl, "SD card free space"=w285:dbl, "CPU Usage"=w290:dbl, "Software Version"=w291:string)
          n130 = Bundle By Name(cluster=T9 {"M2 Heater %"=0.0, "M2 Actuated"=FALSE, "M2 Error"=FALSE, "M2 Thermal Status"=enum."Steady State", "M2 Head State"=enum."Disabled", "M2 Buffer"=0.9999999999999998, "M2 Valve Output"=0.0} ("M2 Cluster"), "M2 Actuated"=w269) -> (w271:T9)
          n131 = property class="Clust (strict)"(reference=w272, "Value"=w271) -> ()  [unwired: 1 in, 2 out]
          n132 = Build Array(w283, w284, w285) -> (w282:dbl[])
          n133 = for {
            tunnel: w282 -> [w294] mode=indexing
            tunnel: [w293] -> w281 mode=indexing
            n134 = Divide(x=w294, y=1000.0) -> (x/y=w293:dbl)
          }
          n135 = Bundle By Name(cluster=T10 {"M1 Heater %"=0.0, "M1 Actuated"=FALSE, "M1 Error"=FALSE, "M1 Thermal Status"=enum."Ramp Up", "M1 Head State"=enum."Disabled", "M1 Buffer"=0.0, "M1 Valve Output"=0.0} ("Value"), "M1 Actuated"=w273) -> (w275:T10)
          n136 = Index Array(array=w281) -> (element #1=w287:dbl, element #2=w288:dbl, element #3=w289:dbl)  [unwired: 3 in]
          n137 = property class="Clust (strict)"(reference=w274, "Value"=w275) -> ()  [unwired: 1 in, 2 out]
          n138 = Bundle By Name(cluster=T8 {"Serial Number"="204300076", "Compressor Hours"=59.65, "SOM Storage(MB)"=243.036, "Memory Available"=353.72, "CPU Usage"=40.953570959266244, "Software Version"="SW Version:CC 21.4.8.1", "SD card free space"=31.886, "Comp Temp"=78.09687988460064, "Sleep Timer"=-1.0, "Sleep"=TRUE, "Boot Up Time"=timestamp(3700144843.654765 s since 1904-01-01)} ("System Cluster"), "Memory Available"=w287, "SOM Storage(MB)"=w288, "SD card free space"=w289, "CPU Usage"=w290, "Software Version"=w291) -> (w277:T8)
          n139 = property class="Clust (strict)"(reference=w278, "Value"=w277) -> ()  [unwired: 1 in, 2 out]
        }
        frame #10 {
          # "Read Network Shared Variables"
          n140 = Concatenate Strings("ni.var.psp://", w299, "/Network Shared Variables/") -> (w297:string)
          n141 = for {
            tunnel: string[] ["AI", "Errors", "TCP Command", "BootupTime", "Output Cluster", "TSD", "DC PS Load Watts", "Event Log", "TCP Connections", "compressor manual frequency control", "Stack Light State", "M1 Values", "TSD Feedback", "M2 Values", "M2 TSD Feedback"] -> [w304] mode=indexing
            tunnel: w297 -> [w305]
            tunnel: w296 -> [w302]
            n142 = Concatenate Strings(w305, w304) -> (w303:string)
            n143 = case shown="\"TSD Feedback\"" w304 {
              tunnel: w303 -> [w309 _ w318 w325 w330 w335 w340 w346 w356 w364 w373 w386 w395]
              tunnel: w302 -> [w308 _ w317 w324 w329 w334 w338 w344 w354 w363 w367 w380 w393]
              frame "Output Cluster" {
                n144 = Unbundle By Name(w308) -> ("M1 Humidity"=w307:refnum<vi>)
                n145 = shared-variable-read(w309, T11 {"Condensing Pressure"=0.0, "Suction Pressure"=0.0, "Bypass steps"=0, "Operating Time"=0.0, "SubCooling"=0.0, "Superheat"=0.0, "M1 Superheat"=0.0, "M2 Superheat"=0.0, "Autotune output"=0.0, "M1 Testing Elapsed Time"=0.0, "M2 Testing Elapsed Time"=0.0, "M1 Valve Control Mode"=0, "System Amps"=0.0, "Compressor Run Time"=0.0, "SD card free Space"=0.0, "Free Memory"=0.0, "M1 Pressure Feedback"=0.0, "M2 Pressure Feedback"=0.0, "Compression Ratio"=0.0, "Serial Number"=0.0, "M1 AC Load V"=0.0, "M1 AC Load W"=0.0, "M1 DC Load W"=0.0, "M1 RH"=0.0, "RH Threshold"=0.0} ("output cluster")) -> (w311:T11)  [unwired: 1 in, 3 out]
                n146 = Unbundle By Name(w311) -> ("RH Threshold"=w313:dbl, "M1 RH"=w312:dbl)
                n147 = Bundle("RH Threshold"=w313, "M1 RH"=w312) -> (w306:cluster{"RH Threshold":dbl, "M1 RH":dbl})  [unwired: 1 in]
                n148 = property class="WFChart (strict)"(reference=w307, "Value"=w306) -> ()  [unwired: 1 in, 2 out]
              }
              frame "TSD" {
              }
              frame "Event Log" {
                n149 = Unbundle By Name(w317) -> ("RT Events"=w314:refnum<vi>)
                n150 = shared-variable-read(w318, T12 [] ("Event Log")) -> (w315:T12)  [unwired: 1 in, 3 out]
                n151 = call "Is Value Changed.vim"("value"=w315) -> ("changed or first call?"=w316:bool)
                n152 = case shown="True" w316 {
                  tunnel: w315 -> [_ w321]
                  tunnel: w314 -> [_ w320]
                  frame False {
                  }
                  frame True {
                    n153 = property class="Arr (strict)"(reference=w320, "Value"=w321) -> ()  [unwired: 1 in, 2 out]
                  }
                }
              }
              frame "Errors" {
                n154 = Unbundle By Name(w324) -> ("Errors"=w323:refnum<vi>)
                n155 = shared-variable-read(w325, string[] [] ("Errors 2")) -> (w322:string[])  [unwired: 1 in, 3 out]
                n156 = property class="Arr (strict)"(reference=w323, "Value"=w322) -> ()  [unwired: 1 in, 2 out]
              }
              frame "TCP Command" {
                n157 = Unbundle By Name(w329) -> ("TCP commands"=w328:refnum<vi>)
                n158 = shared-variable-read(w330, string[] [] ("Errors 2")) -> (w327:string[])  [unwired: 1 in, 3 out]
                n159 = property class="Arr (strict)"(reference=w328, "Value"=w327) -> ()  [unwired: 1 in, 2 out]
              }
              frame "compressor manual frequency control" {
                n160 = Unbundle By Name(w334) -> ("Cascade Compressor controls"=w333:refnum<vi>)
                n161 = shared-variable-read(w335, T13 {"High Stage manual speed control"=FALSE, "Manual High stage frequency"=0.0, "Low Stage manual speed control"=FALSE, "Manual Low Stage frequency"=0.0} ("Cascade Compressor controls")) -> (w332:T13)  [unwired: 1 in, 3 out]
                n162 = property class="Clust (strict)"(reference=w333, "Value"=w332) -> ()  [unwired: 1 in, 2 out]
              }
              frame "Stack Light State" {
                n163 = Unbundle By Name(w338) -> ("RT Status"=w337:refnum<vi>)
                n164 = shared-variable-read(w340, T14."Sleeping Fault" ("Stack light states")) -> (w342:T14)  [unwired: 1 in, 3 out]
                n165 = Format Into String(w342) -> (resulting string=w339:string)  [unwired: 3 in, 1 out]
                n166 = property class="Str"(reference=w337, "Value"=w339) -> ()  [unwired: 1 in, 2 out]
              }
              frame "M1 Values" {
                n167 = Unbundle By Name(w344) -> ("M1 Cluster"=w343:refnum<vi>)
                n168 = shared-variable-read(w346, dbl[] [0.0, 0.0]) -> (w348:dbl[])  [unwired: 1 in, 3 out]
                n169 = Index Array(array=w348) -> (element #1=w350:dbl, element #2=w351:dbl)  [unwired: 2 in]
                n170 = Bundle By Name(cluster=T10 {"M1 Heater %"=0.0, "M1 Actuated"=FALSE, "M1 Error"=FALSE, "M1 Thermal Status"=enum."Steady State", "M1 Head State"=enum."Disabled", "M1 Buffer"=0.9999999999999998, "M1 Valve Output"=0.0} ("M1 Cluster"), "M1 Buffer"=w350, "M1 Valve Output"=w351) -> (w345:T10)
                n171 = property class="Clust (strict)"(reference=w343, "Value"=w345) -> ()  [unwired: 1 in, 2 out]
              }
              frame "M2 Values" {
                n172 = Unbundle By Name(w354) -> ("M2 Cluster"=w353:refnum<vi>)
                n173 = shared-variable-read(w356, dbl[] [0.0, 0.0]) -> (w358:dbl[])  [unwired: 1 in, 3 out]
                n174 = Index Array(array=w358) -> (element #1=w359:dbl, element #2=w360:dbl)  [unwired: 2 in]
                n175 = Bundle By Name(cluster=T9 {"M2 Heater %"=0.0, "M2 Actuated"=FALSE, "M2 Error"=FALSE, "M2 Thermal Status"=enum."Steady State", "M2 Head State"=enum."Disabled", "M2 Buffer"=0.9999999999999998, "M2 Valve Output"=0.0} ("M2 Cluster"), "M2 Buffer"=w359, "M2 Valve Output"=w360) -> (w355:T9)
                n176 = property class="Clust (strict)"(reference=w353, "Value"=w355) -> ()  [unwired: 1 in, 2 out]
              }
              frame "TCP Connections" {
                n177 = Unbundle By Name(w363) -> ("TCP Connections"=w361:refnum<vi>)
                n178 = shared-variable-read(w364, T15 [{"port "=1300, "remote address"="", "Connection timeout ms"=100, "Waiting for connection"=TRUE, "Waiting for Command"=TRUE, "timeout ms"=5000}] ("TCP Connections")) -> (w362:T15)  [unwired: 1 in, 3 out]
                n179 = property class="Arr (strict)"(reference=w361, "Value"=w362) -> ()  [unwired: 1 in, 2 out]
              }
              frame "TSD Feedback" {
                n180 = Unbundle By Name(w367) -> ("M1 Commands"=w366:refnum<vi>)
                n181 = shared-variable-read(w373, FALSE ("data type")) -> (w368:bool)  [unwired: 1 in, 3 out]
                n182 = call "Is Value Changed.vim"("value"=w368) -> ("changed or first call?"=w370:bool)
                n183 = Equal?(x=w368, y=FALSE) -> (x = y?=w369:bool)
                n184 = And(x=w369, y=w370) -> (x .and. y?=w372:bool)
                n185 = case shown="True" w372 {
                  tunnel: w368 -> [w376 _]
                  tunnel: w366 -> [w378 _]
                  frame False {
                    n186 = Bundle By Name(cluster=T16 {"Set Temp"=273.15, "Read Temp"=273.15, "Package"=0, "Bin String"="", "M1 Enable"=TRUE, "TSD"=TRUE} ("Value"), "TSD"=w376) -> (w375:T16)
                    n187 = property on="Property Node" class="Clust (strict)"(reference=w378, "Value"=w375) -> ()  [unwired: 1 in, 2 out]
                  }
                  frame True {
                  }
                }
              }
              frame "M2 TSD Feedback" {
                n188 = Unbundle By Name(w380) -> ("M2 Commands"=w379:refnum<vi>)
                n189 = shared-variable-read(w386, FALSE ("data type")) -> (w381:bool)  [unwired: 1 in, 3 out]
                n190 = call "Is Value Changed.vim"("value"=w381) -> ("changed or first call?"=w383:bool)
                n191 = Equal?(x=w381, y=FALSE) -> (x = y?=w382:bool)
                n192 = And(x=w382, y=w383) -> (x .and. y?=w385:bool)
                n193 = case shown="False" w385 {
                  tunnel: w381 -> [w389 _]
                  tunnel: w379 -> [w391 _]
                  frame False {
                    n194 = Bundle By Name(cluster=T16 {"Set Temp"=273.15, "Read Temp"=273.15, "Package"=0, "Bin String"="", "M1 Enable"=TRUE, "TSD"=TRUE} ("Value"), "TSD"=w389) -> (w388:T16)
                    n195 = property on="Property Node" class="Clust (strict)"(reference=w391, "Value"=w388) -> ()  [unwired: 1 in, 2 out]
                  }
                  frame True {
                  }
                }
              }
              frame "BootupTime", Default {
                n196 = Unbundle By Name(w393) -> ("System Cluster"=w392:refnum<vi>)
                n197 = shared-variable-read(w395, timestamp(0 s since 1904-01-01)) -> (w398:timestamp)  [unwired: 1 in, 3 out]
                n198 = Bundle By Name(cluster=T8 {"Serial Number"="204300076", "Compressor Hours"=59.65, "SOM Storage(MB)"=243.036, "Memory Available"=353.72, "CPU Usage"=40.953570959266244, "Software Version"="SW Version:CC 21.4.8.1", "SD card free space"=31.886, "Comp Temp"=78.09687988460064, "Sleep Timer"=-1.0, "Sleep"=TRUE, "Boot Up Time"=timestamp(3700144843.654765 s since 1904-01-01)} ("System Cluster"), "Boot Up Time"=w398) -> (w394:T8)
                n199 = property class="Clust (strict)"(reference=w392, "Value"=w394) -> ()  [unwired: 1 in, 2 out]
              }
            }
          }
        }
        frame #11 {
          # "Visibility of Controls (Continue~~~~~)"
          n200 = Unbundle By Name(w410) -> ("M1 Safe Temp and Head State"=w408:refnum<vi>, "M1 Power Drive"=w407:refnum<vi>)
          n201 = Unbundle By Name(w405) -> ("Piston Settings.Diameter (mm)"=w406:dbl, "Safe Temps.Enabled"=w402:bool)
          n202 = Unbundle By Name(w411) -> ("Safe Temp"=w401:bool, "Head State"=w409:u16)
          n203 = And(x=w402, y=w401) -> (x .and. y?=w399:bool)
          n204 = Equal To 0?(x=w409) -> (x = 0?=w404:bool)
          n205 = Greater Than 0?(x=w406) -> (x > 0?=w403:bool)
          n206 = And(x=w403, y=w399) -> (x .and. y?=w400:bool)
          n207 = property class="Bool (strict)"(reference=w407, "Visible"=w400) -> ()  [unwired: 1 in, 2 out]
          n208 = property class="Bool (strict)"(reference=w408, "Visible"=w399, "Value"=w404) -> ()  [unwired: 1 in, 2 out]
        }
        frame #12 {
          # "Visibility of Controls (Continue~~~~~)"
          n209 = Unbundle By Name(w424) -> ("M2 Safe Temp and Head State"=w422:refnum<vi>, "M2 Power Drive"=w421:refnum<vi>)
          n210 = Unbundle By Name(w419) -> ("Piston Settings.Diameter (mm)"=w420:dbl, "Safe Temps.Enabled"=w416:bool)
          n211 = Unbundle By Name(w412) -> ("Safe Temp"=w415:bool, "Head State"=w423:u16)
          n212 = And(x=w416, y=w415) -> (x .and. y?=w413:bool)
          n213 = Equal To 0?(x=w423) -> (x = 0?=w418:bool)
          n214 = Greater Than 0?(x=w420) -> (x > 0?=w417:bool)
          n215 = And(x=w417, y=w413) -> (x .and. y?=w414:bool)
          n216 = property class="Bool (strict)"(reference=w421, "Visible"=w414) -> ()  [unwired: 1 in, 2 out]
          n217 = property class="Bool (strict)"(reference=w422, "Visible"=w413, "Value"=w418) -> ()  [unwired: 1 in, 2 out]
        }
        frame #13 {
          w428 = refnum<vi> refnum  # Numeric
          n218 = Unbundle By Name(w431) -> ("Thermal Info"=w430:refnum<vi>)  [unwired: 1 out]
          n219 = Unbundle By Name(w437) -> ("System Settings.Cascade"=w435:bool)
          n220 = Unbundle By Name(w438) -> ("Compressor Amps"=w433:dbl, "Power On Off"=w434:bool)
          n221 = Round To Nearest(number=w433) -> (nearest integer value=w436:dbl)
          n222 = Not Equal To 0?(x=w436) -> (x != 0?=w432:bool)
          n223 = And(x=w432, y=w434) -> (x .and. y?=w425:bool)
          n224 = property class="Clust (strict)"(reference=w430) -> ("Controls[]"=w427:refnum<vi>[])  [unwired: 1 in, 2 out]
          n225 = And(x=w434, y=w435) -> ()  [unwired: 1 out]
          n226 = Index Array(array=w427) -> (element #1=w429:refnum<vi>)  [unwired: 4 in, 3 out]
          n227 = To More Specific Class(target class=w428, reference=w429) -> (specific class reference=w426:refnum<vi>)  [unwired: 1 in, 1 out]
          n228 = property class="Num"(reference=w426, "Visible"=w425) -> ()  [unwired: 1 in, 2 out]
        }
      }
    }
    frame Error {
    }
  }
  "error out" <- w3
  "Cobra GUI out" <- w1
